vi "LOGIC_WriteDCSFrames.vi"(1 "log file":path, 2 "frames to display":T1, 3 "unscramble ptr":u64, 4 "write to disk":bool=TRUE, 5 "reset and expo bpp":u8=16, 6 "TotalPixels":u32, 7 "error in (no error)":errorcluster, 8 "image name":string, 9 "frames to write":T1, 10 "image ptrs (reset - expo)":u64[](array[numeric])) -> (0 "error out":errorcluster)   [LabVIEW 2016]
uses:
  Common/public/vis/CMN_FVAR_action.ctl
  LOGIC_gbls.vi
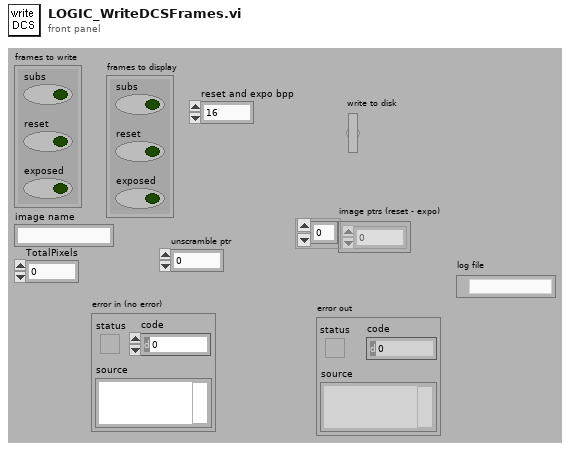
[diagram p1: front panel]
types:
  T1 = cluster{"subs":bool, "reset":bool, "exposed":bool}
  T2 = typedef "CMN_FVAR_action.ctl" = enum16{"read", "write"}
  T3 = typedef "DatabaseHand_RefNum.ctl" = refnum<vi>
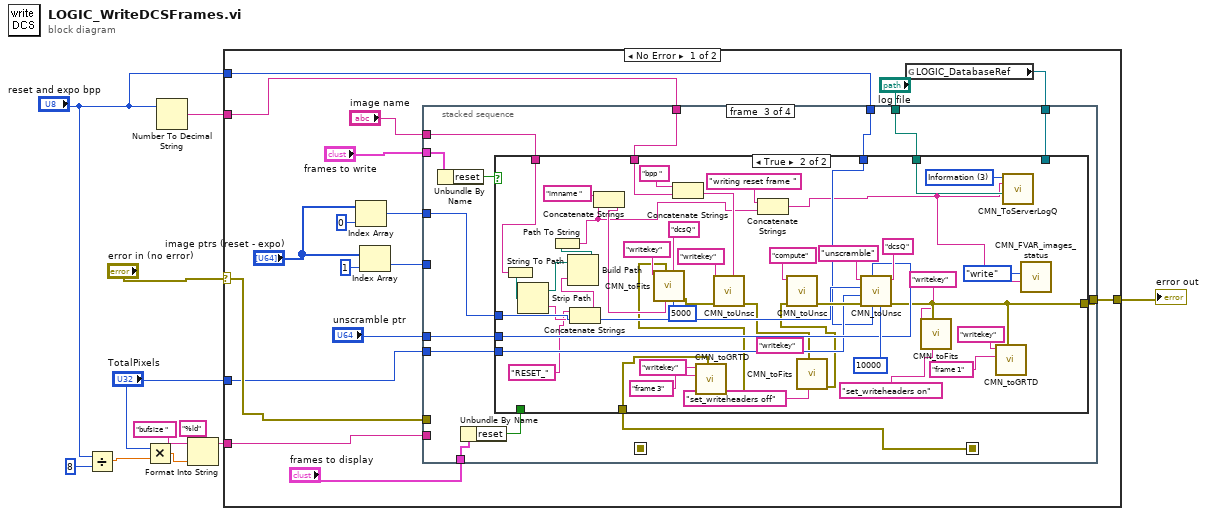
[diagram p0: block diagram]
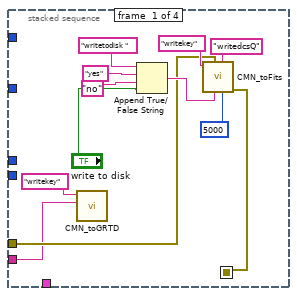
[diagram p2: hidden frame]
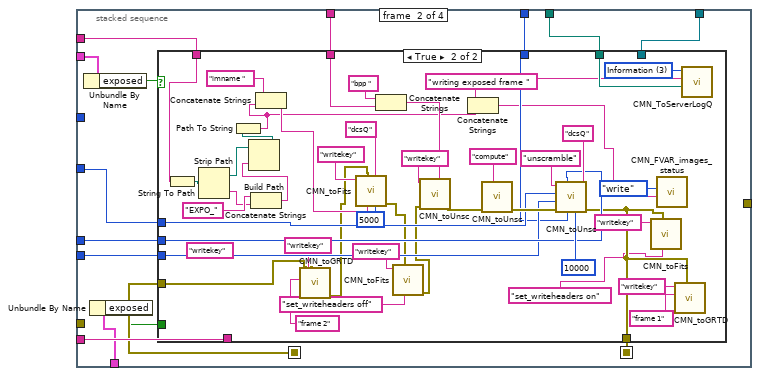
[diagram p3: hidden frame]
diagram:
  (unwired) "%ld" ("Format String")
  n1 = Divide(x="reset and expo bpp", y=u8 8) -> (x/y=w4:dbl)
  n2 = Multiply(x="TotalPixels", y=w4) -> (x*y=w7:dbl)
  n3 = Number To Decimal String(number="reset and expo bpp") -> (decimal integer string=w9:string)  [unwired: 1 out]
  n4 = Format Into String(initial string="bufsize " ("Command"), w7) -> (resulting string=w6:string)  [unwired: 2 in, 1 out]
  n5 = case shown="No Error" "error in (no error)" {
    selector: "error in (no error)" -> [w20 w160]
    tunnel: [w21 w160] -> w1
    tunnel: w9 -> [w19 _]
    tunnel: "TotalPixels" -> [w18 _]
    tunnel: w6 -> [w17 _]
    tunnel: "reset and expo bpp" -> [w16 _]
    frame No Error {
      n6 = Index Array(array="image ptrs (reset - expo)", index=0 ("Index")) -> (element=w23:u64)
      n7 = Index Array(array="image ptrs (reset - expo)", index=1 ("Index")) -> (element=w22:u64)
      n8 = global read "LOGIC_gbls.vi" "LOGIC_DatabaseRef"() -> (w11:T3)
      n9 = stacked-sequence {
        seq-local: [w32 _ _ _] -> [_ w46 _ _]
        seq-local: [_ w44 _ _] -> [_ _ w107 _]
        tunnel: "image name" -> [_ w52 w112 _]
        tunnel: "frames to write" -> [_ w54 w114 _]
        tunnel: w18 -> [_ w51 w111 _]
        tunnel: w23 -> [_ _ w104 _]
        tunnel: w22 -> [_ w43 _ _]
        tunnel: w20 -> [w33 _ _ _]
        tunnel: [_ _ w106 _] -> w21
        tunnel: "unscramble ptr" -> [_ w50 w110 _]
        tunnel: w19 -> [_ w49 w105 _]
        tunnel: w17 -> [w29 w48 _ _]
        tunnel: w16 -> [_ w47 w109 _]
        tunnel: "log file" -> [_ w45 w108 _]
        tunnel: "frames to display" -> [_ w42 w103 _]
        tunnel: w11 -> [_ w40 w101 _]
        frame #0 {
          n10 = call "CMN_toGRTD.vi"("argument"=w29, "Command"="writekey") -> ()  [unwired: 6 in, 4 out]
          n11 = Append True/False String(1:"write to disk", 2:"no" ("false string"), 3:"yes" ("true string"), 4:"writetodisk ") -> (0:w38:string)
          n12 = call "CMN_toFits.vi"("ms timeout (-1)"=5000, "response Q"="writedcsQ", "key"=w38, "error in (no error)"=w33, "command"="writekey") -> ("error out"=w32:errorcluster)  [unwired: 3 in, 3 out]
        }
        frame #1 {
          n13 = Unbundle By Name(w54) -> ("exposed"=w53:bool)
          n14 = Unbundle By Name(w42) -> ("exposed"=w41:bool)
          n15 = case shown="True" w53 {
            tunnel: w52 -> [_ w63]
            tunnel: w51 -> [_ w81]
            tunnel: w43 -> [_ w97]
            tunnel: w46 -> [w55 w73]
            tunnel: w50 -> [_ w82]
            tunnel: w49 -> [_ w87]
            tunnel: w48 -> [_ _]
            tunnel: w47 -> [_ w79]
            tunnel: w45 -> [_ w85]
            tunnel: [w55 w66] -> w44
            tunnel: w41 -> [_ _]
            tunnel: w40 -> [_ _]
            frame False {
            }
            frame True {
              w86 = u16 3 items=["command", "imediateReply", "Callback Reply", "Information"] ("type")
              (unwired) "writekey" ("Command")
              w84 = "writing exposed frame " ("image status")
              n16 = String To Path(string=w63) -> (path=w62:path)
              n17 = Strip Path(path=w62) -> (stripped path=w58:path, name=w60:string)
              n18 = Concatenate Strings("EXPO_" ("Substring"), w60) -> (w59:string)
              n19 = Build Path(base path=w58, name or relative path=w59) -> (appended path=w57:path)
              n20 = Path To String(path=w57) -> (string=w56:string)
              n21 = Concatenate Strings("imname " ("Substring"), w56) -> (w80:string)
              n22 = call "CMN_toGRTD.vi"("error in (no error)"=w73, "argument"="frame 2", "Command"="writekey") -> ("error out"=w78:errorcluster)  [unwired: 5 in, 3 out]
              n23 = call "CMN_toFits.vi"("ms timeout (-1)"=5000, "response Q"="dcsQ", "key"=w80, "error in (no error)"=w78, "command"="writekey") -> ("error out"=w70:errorcluster)  [unwired: 3 in, 3 out]
              n24 = Concatenate Strings("bpp " ("key"), w87) -> (w89:string)
              n25 = call "CMN_toFits.vi"("key"="set_writeheaders off", "error in (no error)"=w70, "command"="writekey") -> ("error out"=w69:errorcluster)  [unwired: 5 in, 3 out]
              n26 = call "CMN_toUnsc.vi"("key"=w89, "error in (no error)"=w69, "command"="writekey") -> ("error out"=w95:errorcluster)  [unwired: 6 in, 2 out]
              n27 = Concatenate Strings(w84, w56) -> (w72:string)
              n28 = call "CMN_toUnsc.vi"("error in (no error)"=w95, "command"="compute") -> ("error out"=w99:errorcluster)  [unwired: 7 in, 2 out]
              n29 = call "CMN_toUnsc.vi"("responseQ"="dcsQ" ("key"), "ms timeout (-1)"=10000, "bpp"=w79, "location 2"=w82, "error in (no error)"=w99, "ele Read"=w81, "location"=w97, "command"="unscramble") -> ("error out"=w66:errorcluster)  [unwired: 1 in, 2 out]
              n30 = call "CMN_toFits.vi"("key"="set_writeheaders on", "error in (no error)"=w66, "command"="writekey") -> ()  [unwired: 5 in, 4 out]
              n31 = call "CMN_FVAR_images_status.vi"("value in"=w72, "action"=CMN_FVAR_action."write") -> ()  [unwired: 9 out]
              n32 = call "CMN_toGRTD.vi"("error in (no error)"=w66, "argument"="frame 1", "Command"="writekey") -> ()  [unwired: 5 in, 4 out]
              n33 = call "CMN_ToServerLogQ.vi"("file"=w85, "string"=w84, "type"=w86) -> ()  [unwired: 3 in, 5 out]
            }
          }
        }
        frame #2 {
          n34 = Unbundle By Name(w114) -> ("reset"=w113:bool)
          n35 = Unbundle By Name(w103) -> ("reset"=w102:bool)
          n36 = case shown="True" w113 {
            tunnel: w112 -> [_ w118]
            tunnel: w111 -> [_ w145]
            tunnel: w104 -> [_ w157]
            tunnel: w107 -> [w115 w132]
            tunnel: w110 -> [_ w146]
            tunnel: w109 -> [_ w144]
            tunnel: w108 -> [_ w150]
            tunnel: [w115 w126] -> w106
            tunnel: w105 -> [_ w140]
            tunnel: w102 -> [_ _]
            tunnel: w101 -> [_ _]
            frame False {
            }
            frame True {
              w151 = u16 3 items=["command", "imediateReply", "Callback Reply", "Information"] ("type")
              (unwired) "writekey" ("command")
              n37 = String To Path(string=w118) -> (path=w123:path)
              n38 = Strip Path(path=w123) -> (stripped path=w121:path, name=w122:string)
              n39 = Concatenate Strings("RESET_" ("Substring"), w122) -> (w117:string)
              n40 = Build Path(base path=w121, name or relative path=w117) -> (appended path=w120:path)
              n41 = Path To String(path=w120) -> (string=w119:string)
              n42 = Concatenate Strings("imname " ("Substring"), w119) -> (w147:string)
              n43 = Concatenate Strings("bpp " ("key"), w140) -> (w139:string)
              n44 = call "CMN_toGRTD.vi"("error in (no error)"=w132, "argument"="frame 3", "Command"="writekey") -> ("error out"=w135:errorcluster)  [unwired: 5 in, 3 out]
              n45 = call "CMN_toFits.vi"("ms timeout (-1)"=5000, "response Q"="dcsQ", "key"=w147, "error in (no error)"=w135, "command"="writekey") -> ("error out"=w142:errorcluster)  [unwired: 3 in, 3 out]
              n46 = call "CMN_toUnsc.vi"("key"=w139, "error in (no error)"=w142, "command"="writekey") -> ("error out"=w128:errorcluster)  [unwired: 6 in, 2 out]
              n47 = Concatenate Strings("writing reset frame " ("image status"), w119) -> (w131:string)
              n48 = call "CMN_toFits.vi"("key"="set_writeheaders off", "error in (no error)"=w128) -> ("error out"=w127:errorcluster)  [unwired: 6 in, 3 out]
              n49 = call "CMN_toUnsc.vi"("error in (no error)"=w127, "command"="compute") -> ("error out"=w159:errorcluster)  [unwired: 7 in, 2 out]
              n50 = call "CMN_toUnsc.vi"("responseQ"="dcsQ", "ms timeout (-1)"=10000, "bpp"=w144, "location 2"=w146, "error in (no error)"=w159, "ele Read"=w145, "location"=w157, "command"="unscramble") -> ("error out"=w126:errorcluster)  [unwired: 1 in, 2 out]
              n51 = call "CMN_toFits.vi"("key"="set_writeheaders on", "error in (no error)"=w126, "command"="writekey") -> ()  [unwired: 5 in, 4 out]
              n52 = call "CMN_toGRTD.vi"("error in (no error)"=w126, "argument"="frame 1", "Command"="writekey") -> ()  [unwired: 5 in, 4 out]
              n53 = call "CMN_ToServerLogQ.vi"("file"=w150, "string"=w131, "type"=w151) -> ()  [unwired: 3 in, 5 out]
              n54 = call "CMN_FVAR_images_status.vi"("value in"=w131, "action"=CMN_FVAR_action."write") -> ()  [unwired: 9 out]
            }
          }
        }
        frame #3 {
        }
      }
    }
    frame Error {
    }
  }
  "error out" <- w1
